vi "Practica2_Semaforo.vi"() -> ()   [LabVIEW 2015]
uses:
  <vilib>/LabVIEW Interface for Arduino/Type Defs/Pin Mode.ctl
  <vilib>/LabVIEW Interface for Arduino/LabVIEW Interface for Arduino.lvlib
panel:
  out "Rojo":bool
  out "Ambar":bool
  out "Verde":bool
  in  "Parar":bool
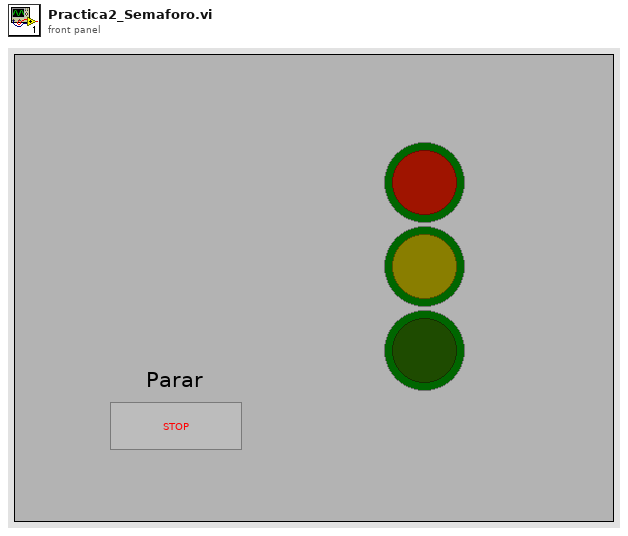
[diagram p1: front panel]
types:
  T1 = typedef "LabVIEW Interface for Arduino.lvlib/Pin Mode.ctl" = enum8{"Input", "Output"}
  T2 = typedef "LabVIEW Interface for Arduino.lvlib/Arduino Resource.ctl" = cluster{"VISA resource":refnum<visa-resource-name>, "Board Type":T3, "Connection Type":enum8{"USB / Serial"}, "Bytes Per Packet (15)":u8}
  T3 = typedef "LabVIEW Interface for Arduino.lvlib/Board Type.ctl" = enum16{"Uno", "Dimuelanove w/Atmega 328", "Mega 2560"}
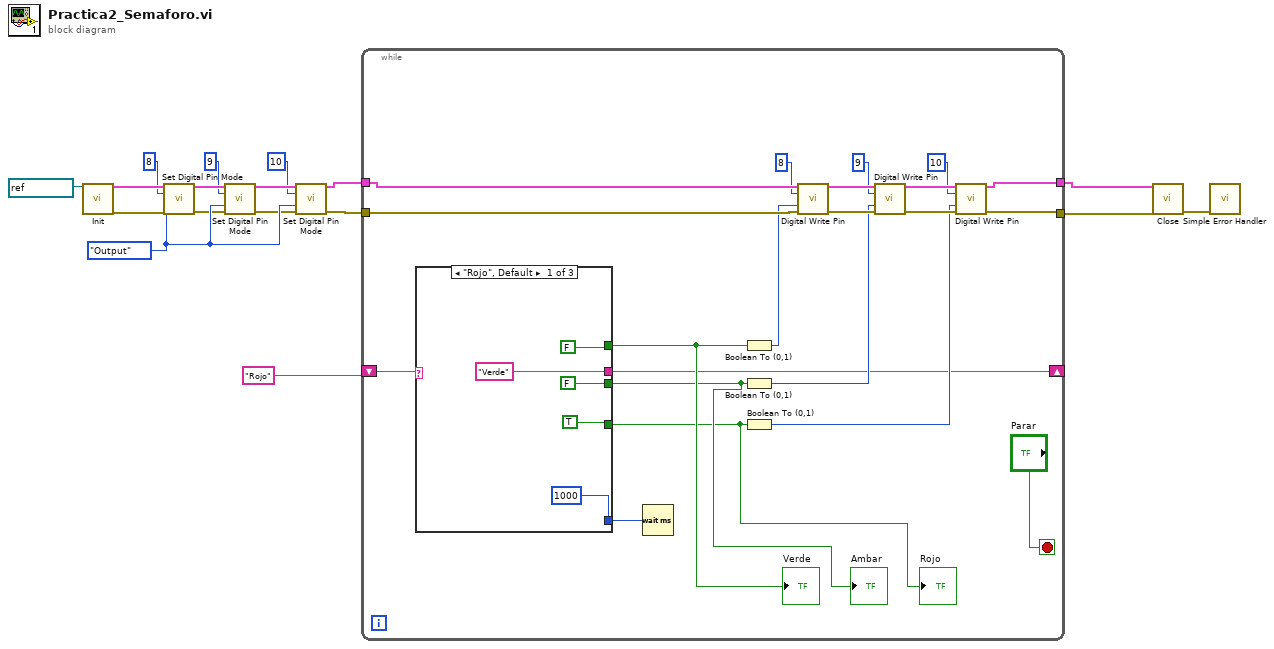
[diagram p0: block diagram]
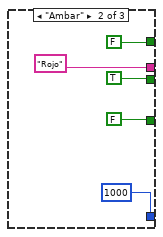
[diagram p2: hidden frame]
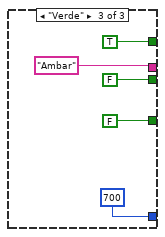
[diagram p3: hidden frame]
diagram:
  w13 = Pin_Mode."Output" ("Pin Mode (Input)")
  n1 = call <vilib>:"Init.vi"("VISA resource"=refnum<visa-resource-name> "COM3") -> ("Arduino Resource"=w16:T2, "error out"=w9:errorcluster)  [unwired: 17 in]
  n2 = call <vilib>:"Set Digital Pin Mode.vi"("Arduino Resource"=w16, "Digital I/O Pin"=u8 8, "Pin Mode (Input)"=w13, "error in"=w9) -> ("Arduino Resource"=w15:T2, "error out"=w8:errorcluster)  [unwired: 10 in]
  n3 = call <vilib>:"Set Digital Pin Mode.vi"("Arduino Resource"=w15, "Digital I/O Pin"=u8 9, "Pin Mode (Input)"=w13, "error in"=w8) -> ("Arduino Resource"=w14:T2, "error out"=w7:errorcluster)  [unwired: 10 in]
  n4 = call <vilib>:"Set Digital Pin Mode.vi"("Arduino Resource"=w14, "Digital I/O Pin"=u8 10, "Pin Mode (Input)"=w13, "error in"=w7) -> ("Arduino Resource"=w4:T2, "error out"=w5:errorcluster)  [unwired: 10 in]
  n5 = while {
    tunnel: w5 -> [w34]
    tunnel: w4 -> [w33]
    tunnel: [w32] -> w3
    tunnel: [w31] -> w2
    shift-right: [w18] -> _
    shift-left: "Rojo" -> [w19]
    stop <- "Parar" stop-if-true
    n6 = case shown="\"Rojo\", Default" w19 {
      tunnel: [u32 1000 ("millisecond timer value") u32 1000 ("millisecond timer value") u32 700 ("millisecond timer value")] -> w27
      tunnel: [FALSE FALSE TRUE] -> w22
      tunnel: [FALSE TRUE FALSE] -> w21
      tunnel: [TRUE FALSE FALSE] -> w20
      tunnel: ["Verde" "Rojo" "Ambar"] -> w18
      frame "Rojo", Default {
      }
      frame "Ambar" {
      }
      frame "Verde" {
      }
    }
    "Verde" <- w22
    "Rojo" <- w20
    "Ambar" <- w21
    n7 = Wait (ms)(milliseconds to wait=w27) -> ()  [unwired: 1 out]
    n8 = Boolean To (0,1)(Boolean=w22) -> (0, 1=w23:i16)
    n9 = Boolean To (0,1)(Boolean=w21) -> (0, 1=w24:i16)
    n10 = Boolean To (0,1)(Boolean=w20) -> (0, 1=w25:i16)
    n11 = call <vilib>:"Digital Write Pin.vi"("Arduino Resource"=w33, "Digital I/O Pin (0)"=u8 8, "Value (0)"=w23, "error in"=w34) -> ("Arduino Resource"=w38:T2, "error out"=w35:errorcluster)  [unwired: 10 in]
    n12 = call <vilib>:"Digital Write Pin.vi"("Arduino Resource"=w38, "Digital I/O Pin (0)"=u8 9, "Value (0)"=w24, "error in"=w35) -> ("Arduino Resource"=w37:T2, "error out"=w36:errorcluster)  [unwired: 10 in]
    n13 = call <vilib>:"Digital Write Pin.vi"("Arduino Resource"=w37, "Digital I/O Pin (0)"=u8 10, "Value (0)"=w25, "error in"=w36) -> ("Arduino Resource"=w31:T2, "error out"=w32:errorcluster)  [unwired: 10 in]
  }
  n14 = call <vilib>:"Close.vi"("Arduino Resource"=w2, "error in"=w3) -> ("error out"=w17:errorcluster)  [unwired: 13 in]
  n15 = call <vilib>:"Simple Error Handler.vi"("error in (no error)"=w17) -> ()  [unwired: 4 in, 5 out]
